vi "initialize_instruments (SubVI).vi"(2 "Run thetaZ?":bool, 3 "Run thetaY?":bool, 4 "Use synth?":bool) -> (0 "tilt stage config":T2, 1 "synth cluster":T1)   [LabVIEW 2016]
uses:
  C:/Users/UsphereLab/Documents/GitHub/Optlev/LabView Code/Tilt Stage/CmdLib.dll
  Tilt Stage/CmdLib.dll
  <instrlib>/Agilent 33XXX Series/Agilent 33XXX Series.lvlib
panel:
  in  "tilt stage config 2":T2
  in  "Y error in (no error)":errorcluster
  in  "Z error in (no error)":errorcluster
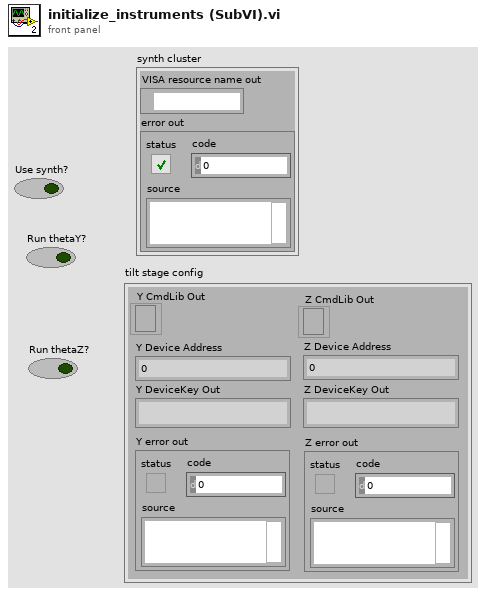
[diagram p1: front panel]
types:
  T1 = cluster{"VISA resource name out":refnum<visa-resource-name>, "error out":errorcluster}
  T2 = cluster{"Y error out":errorcluster, "Y CmdLib Out":refnum<k24>, "Y Device Address":i32, "Y DeviceKey Out":string, "Z error out":errorcluster, "Z CmdLib Out":refnum<k24>, "Z Device Address":i32, "Z DeviceKey Out":string}
  T3 = cluster{"Baud Rate":u32, "Parity":u16, "Data Bits":u16, "Flow Control":u16}
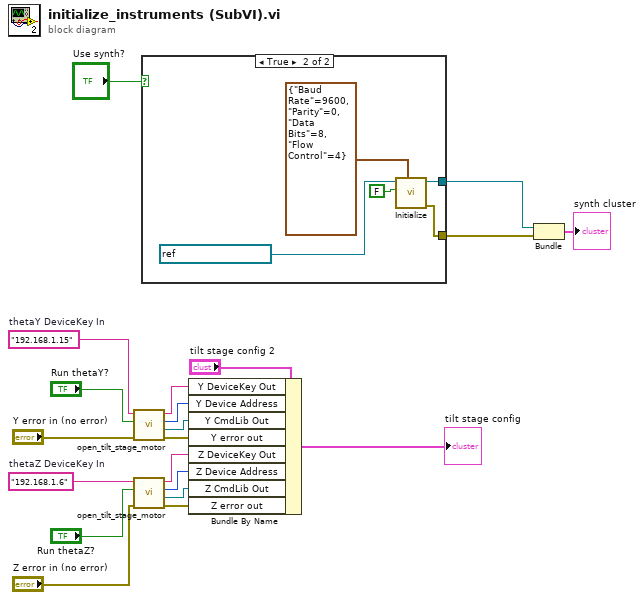
[diagram p0: block diagram]
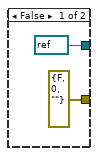
[diagram p2: hidden frame]
diagram:
  w12 = "192.168.1.15"  # thetaY DeviceKey In
  w13 = "192.168.1.6"  # thetaZ DeviceKey In
  n1 = call "open_tilt_stage_motor.vi"("error in (no error)"="Y error in (no error)", "Open device?"="Run thetaY?", "DeviceKey In"=w12) -> ("error out"=w5:errorcluster, "CmdLib Out"=w4:refnum<k24>, "Device Address"=w3:i32, "DeviceKey Out"=w2:string)  [unwired: 1 in]
  n2 = call "open_tilt_stage_motor.vi"("error in (no error)"="Z error in (no error)", "Open device?"="Run thetaZ?", "DeviceKey In"=w13) -> ("error out"=w9:errorcluster, "CmdLib Out"=w8:refnum<k24>, "Device Address"=w7:i32, "DeviceKey Out"=w6:string)  [unwired: 1 in]
  n3 = case shown="True" "Use synth?" {
    tunnel: [refnum<visa-resource-name> refnum ("VISA resource name out") w24] -> w20
    tunnel: [errorcluster {"status"=FALSE, "code"=0, "source"=""} ("error out") w25] -> w19
    frame False {
    }
    frame True {
      n4 = call <instrlib>:"Initialize.vi"("Serial Configuration"=T3 {"Baud Rate"=9600, "Parity"=0, "Data Bits"=8, "Flow Control"=4}, "ID Query (True)"=FALSE, "VISA resource name"=refnum<visa-resource-name> "K-33511B-03409") -> ("error out"=w25:errorcluster, "VISA resource name out"=w24:refnum<visa-resource-name>)  [unwired: 7 in]
    }
  }
  n5 = Bundle By Name(cluster="tilt stage config 2", "Y DeviceKey Out"=w2, "Y Device Address"=w3, "Y CmdLib Out"=w4, "Y error out"=w5, "Z DeviceKey Out"=w6, "Z Device Address"=w7, "Z CmdLib Out"=w8, "Z error out"=w9) -> (→"tilt stage config":T2)
  n6 = Bundle("VISA resource name out"=w20, "error out"=w19) -> (→"synth cluster":T1)  [unwired: 1 in]
